vi "1_Start_Stop.vi"() -> ()   [LabVIEW 2014]
uses:
  <vilib>/DAQmx/create/channels.llb/DAQmx Create Channel (AI-Voltage-Basic).vi
  <vilib>/DAQmx/read.llb/DAQmx Read (Analog DBL 1Chan 1Samp).vi
panel:
  out "Waveform Chart":dbl(graph)
  out "delay":u32
  in  "physical channels":tag
  in  "Use START/STOP Task":bool
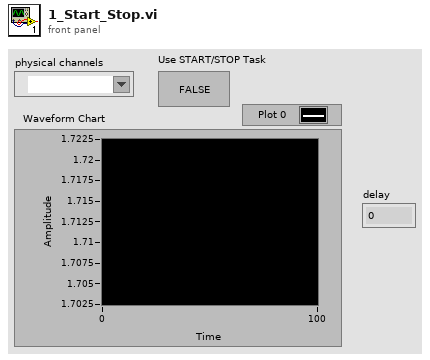
[diagram p1: front panel]
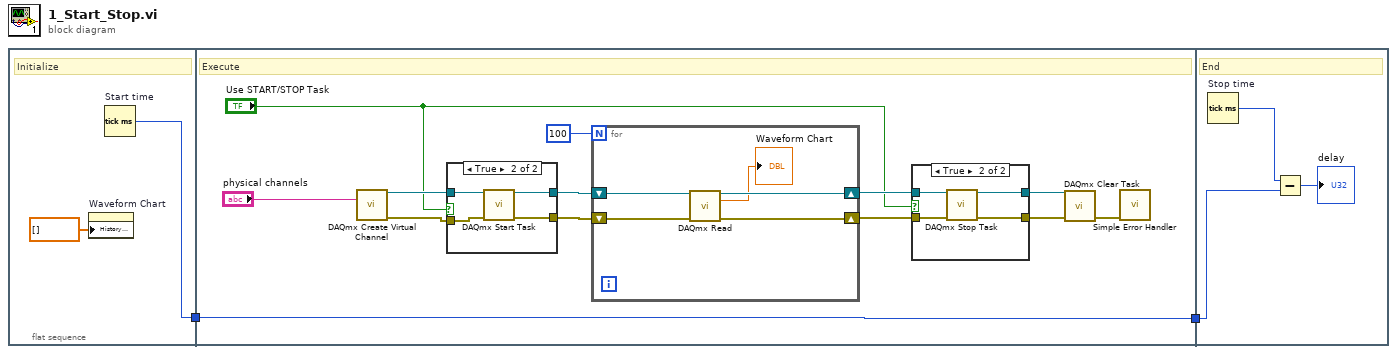
[diagram p0: block diagram]
diagram:
  n1 = flat-sequence {
    tunnel: [w4] -> w2
    tunnel: w2 -> [w6]
    tunnel: [w6] -> w1
    tunnel: w1 -> [w36]
    frame #0 {
      # "Initialize"
      n2 = property on="Waveform Chart" class="WFChart (strict)"("History Data"=dbl[] []) -> ()  [unwired: 2 in, 2 out]
      n3 = Tick Count (ms) "Start time"() -> (millisecond timer value=w4:u32)
    }
    frame #1 {
      # "Execute"
      n4 = call-poly <vilib>:"DAQmx Create Virtual Channel.vi"("physical channels"="physical channels") -> ("task out"=w16:refnum<k21>, "error out"=w15:errorcluster)  [unwired: 13 in]
      n5 = case shown="True" "Use START/STOP Task" {
        tunnel: w16 -> [w30 w33]
        tunnel: w15 -> [w29 w34]
        tunnel: [w30 w32] -> w14
        tunnel: [w29 w31] -> w13
        frame False {
        }
        frame True {
          n6 = call <vilib>:"DAQmx Start Task.vi"("task/channels in"=w33, "error in"=w34) -> ("task out"=w32:refnum<k21>, "error out"=w31:errorcluster)  [unwired: 12 in]
        }
      }
      n7 = for {
        N: 100 -> [_]
        shift-right: [w20] -> w12
        shift-left: w14 -> [w22]
        shift-right: [w19] -> w11
        shift-left: w13 -> [w21]
        n8 = call-poly <vilib>:"DAQmx Read.vi"("task/channels in"=w22, "error in"=w21) -> ("task out"=w20:refnum<k21>, "data"=→"Waveform Chart":dbl, "error out"=w19:errorcluster)  [unwired: 11 in]
      }
      n9 = case shown="True" "Use START/STOP Task" {
        tunnel: w12 -> [w24 w28]
        tunnel: w11 -> [w23 w27]
        tunnel: [w24 w26] -> w10
        tunnel: [w23 w25] -> w9
        frame False {
        }
        frame True {
          n10 = call <vilib>:"DAQmx Stop Task.vi"("task/channels in"=w28, "error in"=w27) -> ("task out"=w26:refnum<k21>, "error out"=w25:errorcluster)  [unwired: 12 in]
        }
      }
      n11 = call <vilib>:"DAQmx Clear Task.vi"("task in"=w10, "error in"=w9) -> ("error out"=w7:errorcluster)  [unwired: 13 in]
      n12 = call <vilib>:"Simple Error Handler.vi"("error in (no error)"=w7) -> ()  [unwired: 4 in, 5 out]
    }
    frame #2 {
      # "End"
      n13 = Tick Count (ms) "Stop time"() -> (millisecond timer value=w37:u32)
      n14 = Subtract(x=w37, y=w36) -> (x-y=→"delay":u32)
    }
  }
